vi "sequence8Digit.vi"(8 "Error In":errorcluster, 11 "Trace Number In":string) -> (0 "Error Out":errorcluster, 3 "Trace Number Out":string)   [LabVIEW 2018]
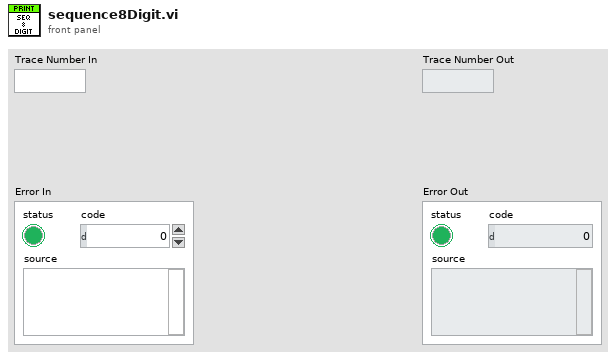
[diagram p1: front panel]
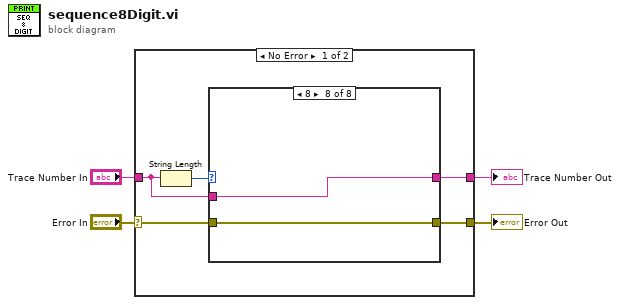
[diagram p0: block diagram]
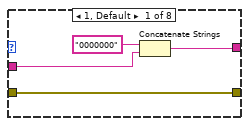
[diagram p2: hidden frame]
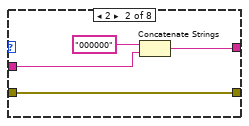
[diagram p3: hidden frame]
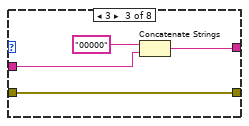
[diagram p4: hidden frame]
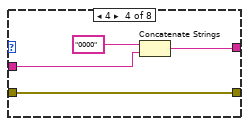
[diagram p5: hidden frame]
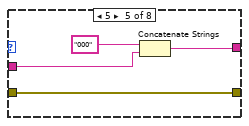
[diagram p6: hidden frame]
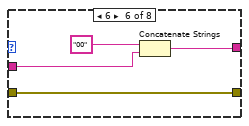
[diagram p7: hidden frame]
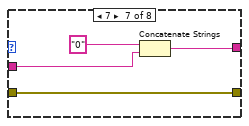
[diagram p8: hidden frame]
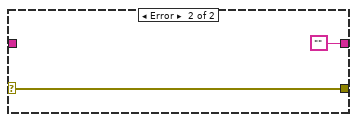
[diagram p9: hidden frame]
diagram:
  n1 = case shown="No Error" "Error In" {
    selector: "Error In" -> [w9 w41]
    tunnel: [w8 w41] -> w3
    tunnel: "Trace Number In" -> [w6 _]
    tunnel: [w5 ""] -> w1
    frame No Error {
      n2 = String Length(string=w6) -> (length=w7:i32)
      n3 = case shown="8" w7 {
        tunnel: w9 -> [w13 w17 w21 w25 w29 w33 w37 w39]
        tunnel: [w13 w17 w21 w25 w29 w33 w37 w39] -> w8
        tunnel: w6 -> [w11 w15 w19 w23 w27 w31 w35 w38]
        tunnel: [w10 w14 w18 w22 w26 w30 w34 w38] -> w5
        frame 1, Default {
          n4 = Concatenate Strings("0000000", w11) -> (w10:string)
        }
        frame 2 {
          n5 = Concatenate Strings("000000", w15) -> (w14:string)
        }
        frame 3 {
          n6 = Concatenate Strings("00000", w19) -> (w18:string)
        }
        frame 4 {
          n7 = Concatenate Strings("0000", w23) -> (w22:string)
        }
        frame 5 {
          n8 = Concatenate Strings("000", w27) -> (w26:string)
        }
        frame 6 {
          n9 = Concatenate Strings("00", w31) -> (w30:string)
        }
        frame 7 {
          n10 = Concatenate Strings("0", w35) -> (w34:string)
        }
        frame 8 {
        }
      }
    }
    frame Error {
    }
  }
  "Trace Number Out" <- w1
  "Error Out" <- w3
